vi "MicrostepCurve.vi"(1 "Enum":enum16{"16", "8"}(ring)) -> (0 "microstepCurve":i32[](array[numeric]))   [LabVIEW 2022 SP3, in "Motorshield.lvlib"]
uses:
  Motorshield.lvlib
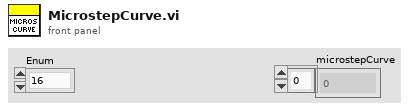
[diagram p1: front panel]
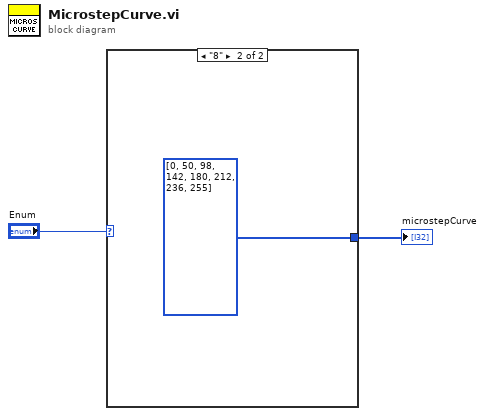
[diagram p0: block diagram]
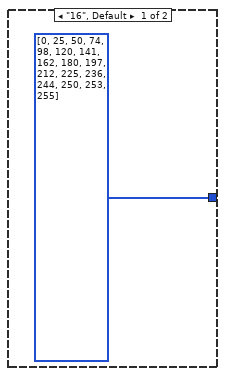
[diagram p2: hidden frame]
diagram:
  n1 = case shown="\"8\"" "Enum" {
    tunnel: [i32[] [0, 25, 50, 74, 98, 120, 141, 162, 180, 197, 212, 225, 236, 244, 250, 253, 255] i32[] [0, 50, 98, 142, 180, 212, 236, 255]] -> w1
    frame "16", Default {
    }
    frame "8" {
    }
  }
  "microstepCurve" <- w1
